vi "ConfigSignal.vi"(8 "Error in":errorcluster, 9 "SampleRate":dbl, 10 "FilterFrequency":dbl, 11 "Signal":refnum<k24>) -> (0 "Error out":errorcluster)   [LabVIEW 2016]
doc: "Configurates the signal according to given parameters. \nIf the signal does not support a filter frequency (e.g. a virtual signal like a calculated channel) NO error will be created here.\nRemarks: To configure the physical device with these settings, you have to use the AssignSignals VI when the signal is configured.\n\nSignal: The signal you want to configurate\nSampleRate: Sample rate that should be used for measurement \nFilterFrequency: Filter frequency to use ( filter type - e.g. Bessel or Butterworth will not be changed!)"
uses:
  C:/Users/CL/Desktop/ZcDAQprj0811/ZcDAQprj/Modules/DAQ-Device/Hardware Drivers/QX/HBM LabVIEW Driver/DLLs/Hbm.Api.Common.dll
  DLLs/Hbm.Api.Common.dll
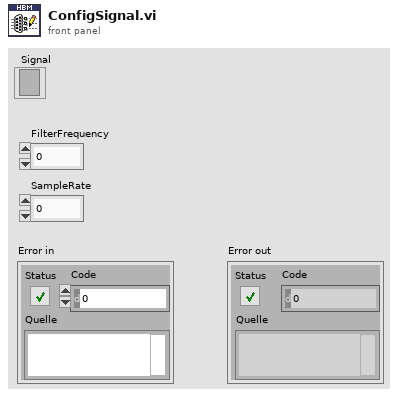
[diagram p1: front panel]
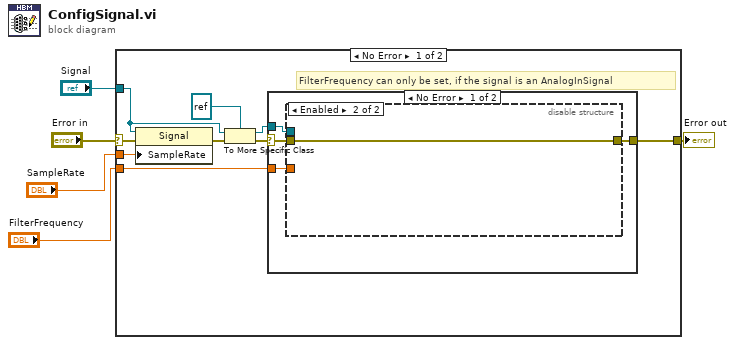
[diagram p0: block diagram]
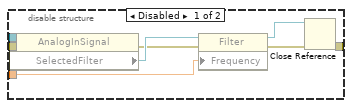
[diagram p2: hidden frame]
diagram:
  n1 = case shown="No Error" "Error in" {
    selector: "Error in" -> [w8 w28]
    tunnel: "Signal" -> [w14 _]
    tunnel: "FilterFrequency" -> [w11 _]
    tunnel: [w10 w28] -> w2
    tunnel: "SampleRate" -> [w9 _]
    frame No Error {
      # "FilterFrequency can only be set, if the signal is an AnalogInSignal"
      n2 = property on="Eigenschaftsknoten" class="Signal"(reference=w14, error in=w8, "SampleRate"=w9) -> (error out=w7:errorcluster)  [unwired: 1 out]
      n3 = To More Specific Class(target class=refnum<k24> refnum (".NET (Referenz)"), reference=w14, error in=w7) -> (specific class reference=w12:refnum<k24>, error out=w13:errorcluster)
      n4 = case shown="No Error" w13 {
        selector: w13 -> [w17 _]
        tunnel: w12 -> [w18 _]
        tunnel: w11 -> [w16 _]
        tunnel: [w15 _] -> w10
        frame No Error {
          n5 = disable-structure shown="Enabled" {
            disable-tunnel: w18 -> [w26 _]
            disable-tunnel: w17 -> [w25 w27]
            disable-tunnel: w16 -> [w24 _]
            disable-tunnel: [w23 w27] -> w15
            frame Disabled {
              n6 = property on="Eigenschaftsknoten" class="AnalogInSignal"(reference=w26, error in=w25) -> (error out=w21:errorcluster, "SelectedFilter"=w22:refnum<k24>)  [unwired: 1 out]
              n7 = property on="Eigenschaftsknoten" class="Filter"(reference=w22, error in=w21, "Frequency"=w24) -> (reference out=w19:refnum<k24>, error out=w20:errorcluster)
              n8 = Close Reference(reference=w19, error in (no error)=w20) -> (error out=w23:errorcluster)
            }
            frame Enabled {
            }
          }
        }
        frame Error {
        }
      }
    }
    frame Error {
    }
  }
  "Error out" <- w2
